vi "WPL_start cdb waveform.vi"(8 "error in (no error)":errorcluster, 10 "t0":timestamp, 11 "WPL Comm in":refnum<class "WPL Comm.lvclass">) -> (0 "error out":errorcluster)   [LabVIEW 2020, in "Internal Comm Classes.lvlib" / "WPL Comm.lvclass"]
uses:
  WPL Comm.lvclass
  WPL Command.ctl
  WPL Comm.lvclass/WPL Comm.ctl
  Convert Q Error to Shutdown Error.vi
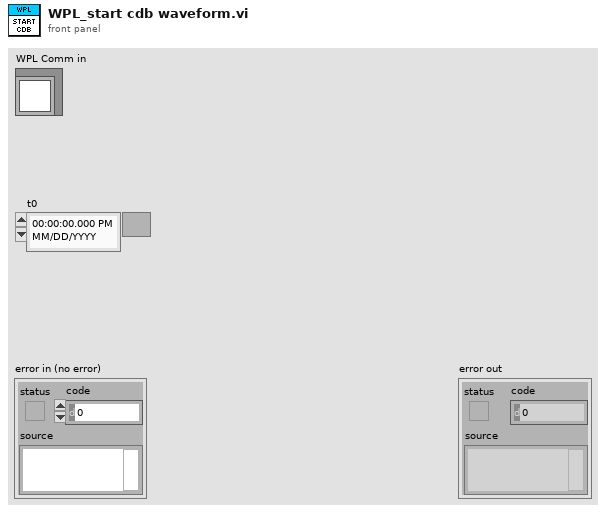
[diagram p1: front panel]
types:
  T1 = typedef "Internal Comm Classes.lvlib/WPL Comm.lvclass/WPL Command.ctl" = enum16{"Register 1D DBL Reader", "Unregister 1D DBL Reader", "Register 1D DBL Writer", "Register 2D DBL Writer", "Unregister 1D DBL Writer", "Unregister 2D DBL Writer", "DBL WFM Start", "WFM 1D DBL Data", "WFM 2D DBL Data", "Shut down", "Handle Error", "Register 1D CDB Reader", "Unregister 1D CDB Reader", "Register 1D CDB Writer", "Unregister 1D CDB Writer", "Register 2D CDB Writer", "Unregister 2D CDB Writer", "WFM 1D CDB Data", "WFM 2D CDB Data", "CDB WFM Start", "Error Shutdown", "Register Streams", "Unregister Streams", "Delete All Streams", "Get WFM DTs", "DBL WFM Multi Start", "CDB WFM Multi Start"}
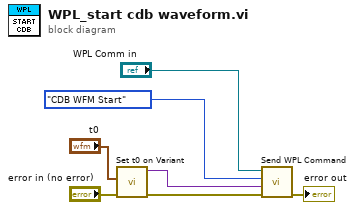
[diagram p0: block diagram]
diagram:
  n1 = call "Set t0 on Variant.vi"("error in (no error)"="error in (no error)", "t0"="t0") -> ("error out"=w6:errorcluster, "Variant out"=w1:variant)  [unwired: 7 in, 1 out]
  n2 = call "Send WPL Command.vi"("error in (no error)"=w6, "Variant"=w1, "Command"=WPL_Command."CDB WFM Start", "WPL Comm"="WPL Comm in") -> ("error out"=→"error out":errorcluster)  [unwired: 6 in, 1 out]
